vi "Task4.vi"() -> ()   [LabVIEW 2020]
panel:
  out "Pulse Time (us)":u16
  out "Pulse Count":i32
  in  "Serial Port":refnum<visa-resource-name>="COM4"
  in  "Voltage":dbl(slide) scale=-100.0..100.0
  in  "stop":bool
  out "RPM":dbl(knob) scale=0.0..200.0
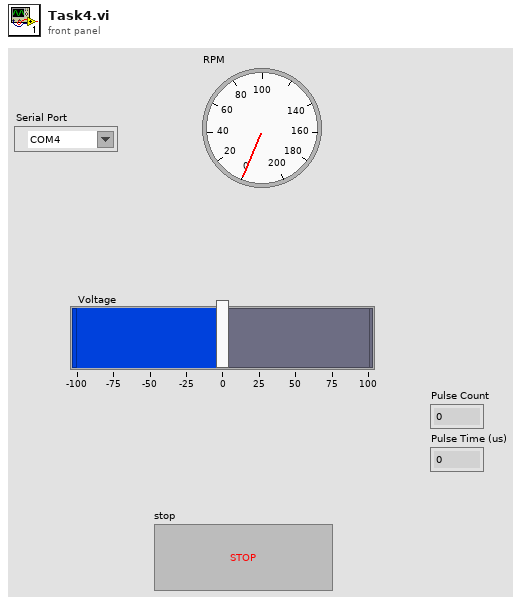
[diagram p1: front panel]
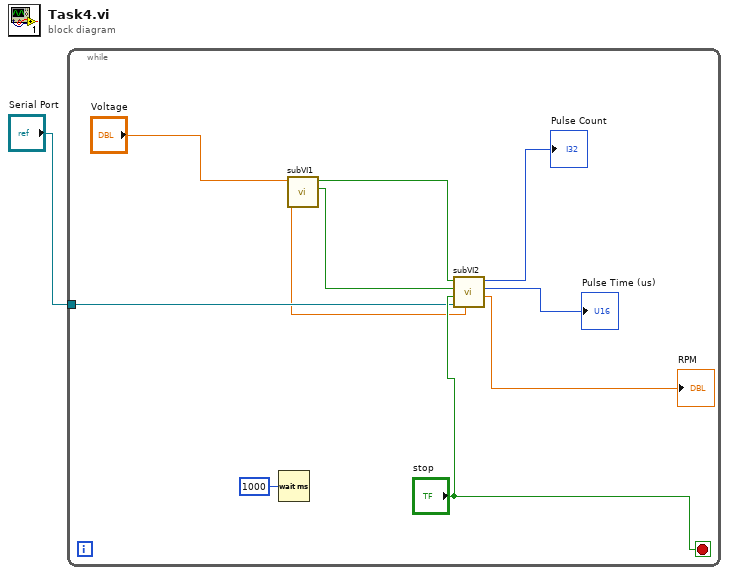
[diagram p0: block diagram]
diagram:
  n1 = while {
    tunnel: "Serial Port" -> [w6]
    stop <- "stop" stop-if-true
    n2 = Wait (ms)(milliseconds to wait=u32 1000) -> ()  [unwired: 1 out]
    n3 = call "subVI1.vi"("Numeric"="Voltage") -> ("B"=w8:bool, "A"=w9:bool, "x/y"=w2:dbl)  [unwired: 8 in]
    n4 = call "subVI2.vi"("Duty Cycle (0-1)"=w2, "Serial Port"=w6, "stop"="stop", "B"=w8, "A"=w9) -> ("x/y"=→"RPM":dbl, "Pulse Time (us)"=→"Pulse Time (us)":u16, "Pulse Count"=→"Pulse Count":i32)  [unwired: 4 in]
  }
